vi "APS get sscnet servo alarm.vi"(8 "error in (no error)":errorcluster caption="错误输入（无错误）", 9 "Alarm_Detail":i32, 10 "Alarm_No":i32, 11 "Axis_ID":i32) -> (0 "error out":errorcluster caption="错误输出", 1 "Alarm_Detail out":i32, 2 "Alarm_No out":i32, 3 "function return":i32)   [LabVIEW 2011, in "APS168.lvlib"]
doc: "I32 FNTYPE APS_get_sscnet_servo_alarm( I32 Axis_ID, I32 *Alarm_No, I32 *Alarm_Detail );"
uses:
  APS168.lvlib
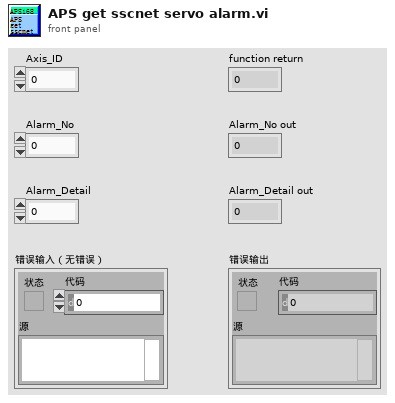
[diagram p1: front panel]
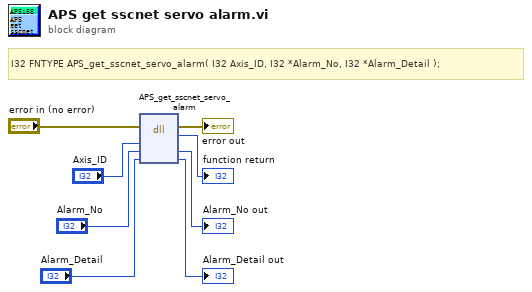
[diagram p0: block diagram]
diagram:
  # "I32 FNTYPE APS_get_sscnet_servo_alarm( I32 Axis_ID, I32 *Alarm_No, I32 *Alarm_Detail );"
  n1 = dll-call lib="PTH1Labs E软件ADLINK 204CAPS_1_7_1_LIB line 连续运动204APS168.*" fn="APS_get_sscnet_servo_alarm"(error in="error in (no error)", "Axis_ID"="Axis_ID", "Alarm_No"="Alarm_No", "Alarm_Detail"="Alarm_Detail") -> (error out=→"error out":errorcluster, →"function return":i32, "Alarm_No"=→"Alarm_No out":i32, "Alarm_Detail"=→"Alarm_Detail out":i32)  [unwired: 3 in, 1 out]
